vi "Module Type.vi"(11 "Messaging Client in":refnum<class "Messaging Server Client.lvclass">) -> (2 "Module Type":string)   [LabVIEW 2020, in "Volatus.lvlib" / "Messaging Server Client.lvclass"]
uses:
  Messaging Server Client.lvclass
  Messaging Server Client.lvclass/Messaging Server Client.ctl
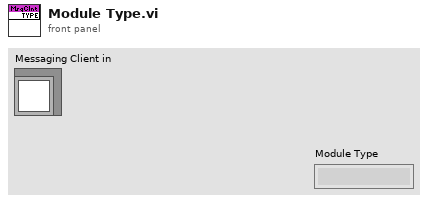
[diagram p1: front panel]
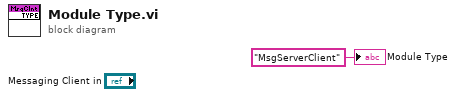
[diagram p0: block diagram]
diagram:
  "Module Type" <- "MsgServerClient" ("Module Type")
